vi "Arms SSO.vi"(11 "Arms Actuators In":T1) -> ()   [LabVIEW 2014]
uses:
  Arms SS Typedef.ctl
  <vilib>/Rock Robotics/WPI/Solenoid/WPI_SolenoidValue.ctl
  Global Variables/Refnum Names.vi
  <vilib>/Rock Robotics/WPI/Solenoid/WPI_SolenoidSetEnum.vi
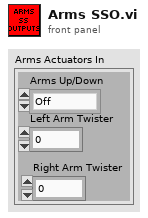
[diagram p1: front panel]
types:
  T1 = typedef "Arms SS Typedef.ctl" = cluster{"Arms Up/Down":T2, "Left Arm Twister":dbl, "Right Arm Twister":dbl}
  T2 = typedef "WPI_SolenoidValue.ctl" = enum16{"Off", "On", "Forward", "Reverse"}
  T3 = typedef "WPI_SolenoidDevRef.ctl" = cluster{"DevStatus":errorcluster, "Pneumatics Control Module":u8, "Forward Solenoid Channel":T4, "Reverse Solenoid Channel":T4}
  T4 = typedef "WPI_SolenoidChannel.ctl" = enum8{"Solenoid 0", "Solenoid 1", "Solenoid 2", "Solenoid 3", "Solenoid 4", "Solenoid 5", "Solenoid 6", "Solenoid 7", "Invalid"}
  T5 = typedef "WPI_ServoDeviceRef.ctl" = cluster{"DeviceStatus":errorcluster, "Controller":T6, "PWM Channel":T7, "DeadBand":T8}
  T6 = typedef "FPGA_TypedefDigitalModule.ctl" = enum16{"Controller 1"}
  T7 = typedef "FPGA_DIOPWMChannel.ctl" = enum8{"PWM 0", "PWM 1", "PWM 2", "PWM 3", "PWM 4", "PWM 5", "PWM 6", "PWM 7", "PWM 8", "PWM 9", "PWM MXP 0", "PWM MXP 1", "PWM MXP 2", "PWM MXP 3", "PWM MXP 4", "PWM MXP 5", "PWM MXP 6", "PWM MXP 7", "PWM MXP 8", "PWM MXP 9", "Invalid"}
  T8 = typedef "WPI_PWMDeadband.ctl" = cluster{"Name":string, "maxPositivePwm":i32, "minPositivePwm":i32, "centerPwm":i32, "maxNegativePwm":i32, "minNegativePwm":i32, "angularRange":u16}
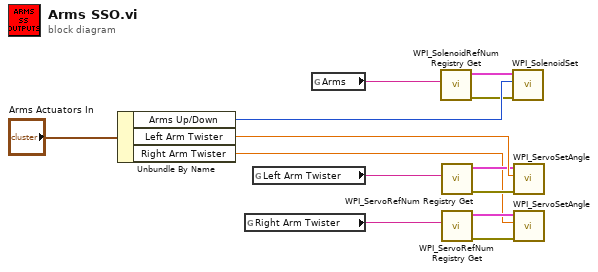
[diagram p0: block diagram]
diagram:
  n1 = Unbundle By Name("Arms Actuators In") -> ("Arms Up/Down"=w11:T2, "Left Arm Twister"=w12:dbl, "Right Arm Twister"=w1:dbl)
  n2 = global read "Refnum Names.vi" "Right Arm Twister"() -> (w2:string)
  n3 = global read "Refnum Names.vi" "Left Arm Twister"() -> (w10:string)
  n4 = global read "Refnum Names.vi" "Arms"() -> (w5:string)
  n5 = call <vilib>:"WPI_SolenoidRefNum Registry Get.vi"("refnum name"=w5) -> ("error out"=w7:errorcluster, "SolenoidDevRef"=w6:T3)  [unwired: 9 in]
  n6 = call <vilib>:"WPI_ServoRefNum Registry Get.vi"("refnum name"=w10) -> ("error out"=w8:errorcluster, "ServoDeviceRef"=w9:T5)  [unwired: 9 in]
  n7 = call <vilib>:"WPI_ServoRefNum Registry Get.vi"("refnum name"=w2) -> ("error out"=w3:errorcluster, "ServoDeviceRef"=w4:T5)  [unwired: 9 in]
  n8 = call-poly <vilib>:"WPI_SolenoidSet.vi"("error in (no error)"=w7, "Value"=w11, "SolenoidDevRef"=w6) -> ()  [unwired: 7 in, 2 out]
  n9 = call <vilib>:"WPI_ServoSetAngle.vi"("error in (no error)"=w8, "Angle"=w12, "ServoDeviceRef"=w9) -> ()  [unwired: 7 in, 2 out]
  n10 = call <vilib>:"WPI_ServoSetAngle.vi"("error in (no error)"=w3, "Angle"=w1, "ServoDeviceRef"=w4) -> ()  [unwired: 7 in, 2 out]
